vi "Setup Fast F Sweep.vi"(4 "TO, ms":u32=100, 5 "Retry on TO":bool, 7 "Generate F array":bool=TRUE, 8 "error in":errorcluster, 11 "RUS settings in":T1={"NI-DAQ lockin settings"={"Samples per sine wave"=0, "Sine waves per freq step"=0, "Output Representation"=enum."Real/Imaginary", "Low-pass filter"=enum."Butterworth", "Ranges and couplings "=[]}, "Fast swep settings"={"Update rate (Hz)"=250.0, "Start F, Hz"=200000.0, "Stop F"=1700000.0, "Number of points"=30000, "Amplitude"=2.1, "Init&amplitude"=TRUE, "IF"=1000.0, "Time constant"=0.1}, "Pre-sweep delay, s"=0.0, "Lockin mode"=enum."NI-DAQ", "SR Lockin"="GPIB0::10::INSTR", "DAQmx Device"="Dev3", "Clock Multiplier"=64, "Fast Sweep Data Out"={"DO clock task"="", "DO task"="", "Update clock task"="", "DAQ lockin task"="", "Pre-sweep counter task"=""}, "Lockin Range, V"=0.0, "F Array"=[], "Freq. update clock terminal"="", "DO Clock Rate (Hz)"=5000000.0, "ADC clock terminal"="/PFI4", "Pre-sweep counter terminal"="", "Samples per read"=10, "DO clock terminal"="", "Pre-sweep points"=0, "F points per write"=1000, "Total sweep time, s"=0.0, "Initial SYNTH phase"=0.0, "Record IF"=FALSE, "Save data settings"={"Save data"=TRUE, "Data Root Path"=path "", "File Prefix"="", "File Format"=enum."ASCII", "Save column names"=TRUE, "File Comments"="<Description of the current file>", "User/Prj"="<User Name/Project Description>"}, "Data file path"=path "", "New data user event"=refnum, "Stop user event"=refnum, "Number of channels"=1, "Auto-phase"=FALSE, "RP Transeiver"=refnum} {"Lockin Range, V" format="%#_6e"; "Fast swep settings"."IF" format="%#_6p"; "Fast swep settings"."Amplitude" min=0.0 max=2.5; "Fast swep settings"."Number of points" format="%.0p"; "Fast swep settings"."Stop F" format="%#_6p"; "Fast swep settings"."Start F, Hz" format="%#_6p"; "Fast swep settings"."Update rate (Hz)" format="%0.2f"; "NI-DAQ lockin settings"."Ranges and couplings"."Coupling" items=["default"=-1, "RSE"=10083, "NRSE"=10078, "Differential"=10106, "Pseudodifferential"=12529]}) -> (0 "error out":errorcluster, 1 "DO task setup time":u32, 3 "RUS settings out":T1={"NI-DAQ lockin settings"={"Samples per sine wave"=0, "Sine waves per freq step"=0, "Output Representation"=enum."Real/Imaginary", "Low-pass filter"=enum."Butterworth", "Ranges and couplings "=[]}, "Fast swep settings"={"Update rate (Hz)"=250.0, "Start F, Hz"=200000.0, "Stop F"=1700000.0, "Number of points"=30000, "Amplitude"=2.1, "Init&amplitude"=TRUE, "IF"=1000.0, "Time constant"=0.1}, "Pre-sweep delay, s"=0.0, "Lockin mode"=enum."NI-DAQ", "SR Lockin"="GPIB0::10::INSTR", "DAQmx Device"="Dev3", "Clock Multiplier"=64, "Fast Sweep Data Out"={"DO clock task"="", "DO task"="", "Update clock task"="", "DAQ lockin task"="", "Pre-sweep counter task"=""}, "Lockin Range, V"=0.0, "F Array"=[], "Freq. update clock terminal"="", "DO Clock Rate (Hz)"=5000000.0, "ADC clock terminal"="/PFI4", "Pre-sweep counter terminal"="", "Samples per read"=10, "DO clock terminal"="", "Pre-sweep points"=0, "F points per write"=1000, "Total sweep time, s"=0.0, "Initial SYNTH phase"=0.0, "Record IF"=FALSE, "Save data settings"={"Save data"=TRUE, "Data Root Path"=path "", "File Prefix"="", "File Format"=enum."ASCII", "Save column names"=TRUE, "File Comments"="<Description of the current file>", "User/Prj"="<User Name/Project Description>"}, "Data file path"=path "", "New data user event"=refnum, "Stop user event"=refnum, "Number of channels"=1, "Auto-phase"=FALSE, "RP Transeiver"=refnum} {"Lockin Range, V" format="%#_6e"; "Fast swep settings"."IF" format="%#_6p"; "Fast swep settings"."Amplitude" min=0.0 max=2.5; "Fast swep settings"."Number of points" format="%.0p"; "Fast swep settings"."Stop F" format="%#_6p"; "Fast swep settings"."Start F, Hz" format="%#_6p"; "Fast swep settings"."Update rate (Hz)" format="%0.2f"; "NI-DAQ lockin settings"."Ranges and couplings"."Coupling" items=["default"=-1, "RSE"=10083, "NRSE"=10078, "Differential"=10106, "Pseudodifferential"=12529]})   [LabVIEW 2016]
uses:
  Controls/Lockin mode.ctl
  NHMFL_Core/Libraries/Red Pitaya/RP Core/RP Transceiver/RP Transceiver.lvclass
  Controls/Sweep settings.ctl
  Controls/RUS NI-DAQ Lockin Settings.ctl
  Controls/RUS settings.ctl
  NHMFL_Core/Libraries/File/Controls/File formats.ctl
  NHMFL_Core/Libraries/File/Controls/Save data settings.ctl
panel:
  out "F1 out time":u32
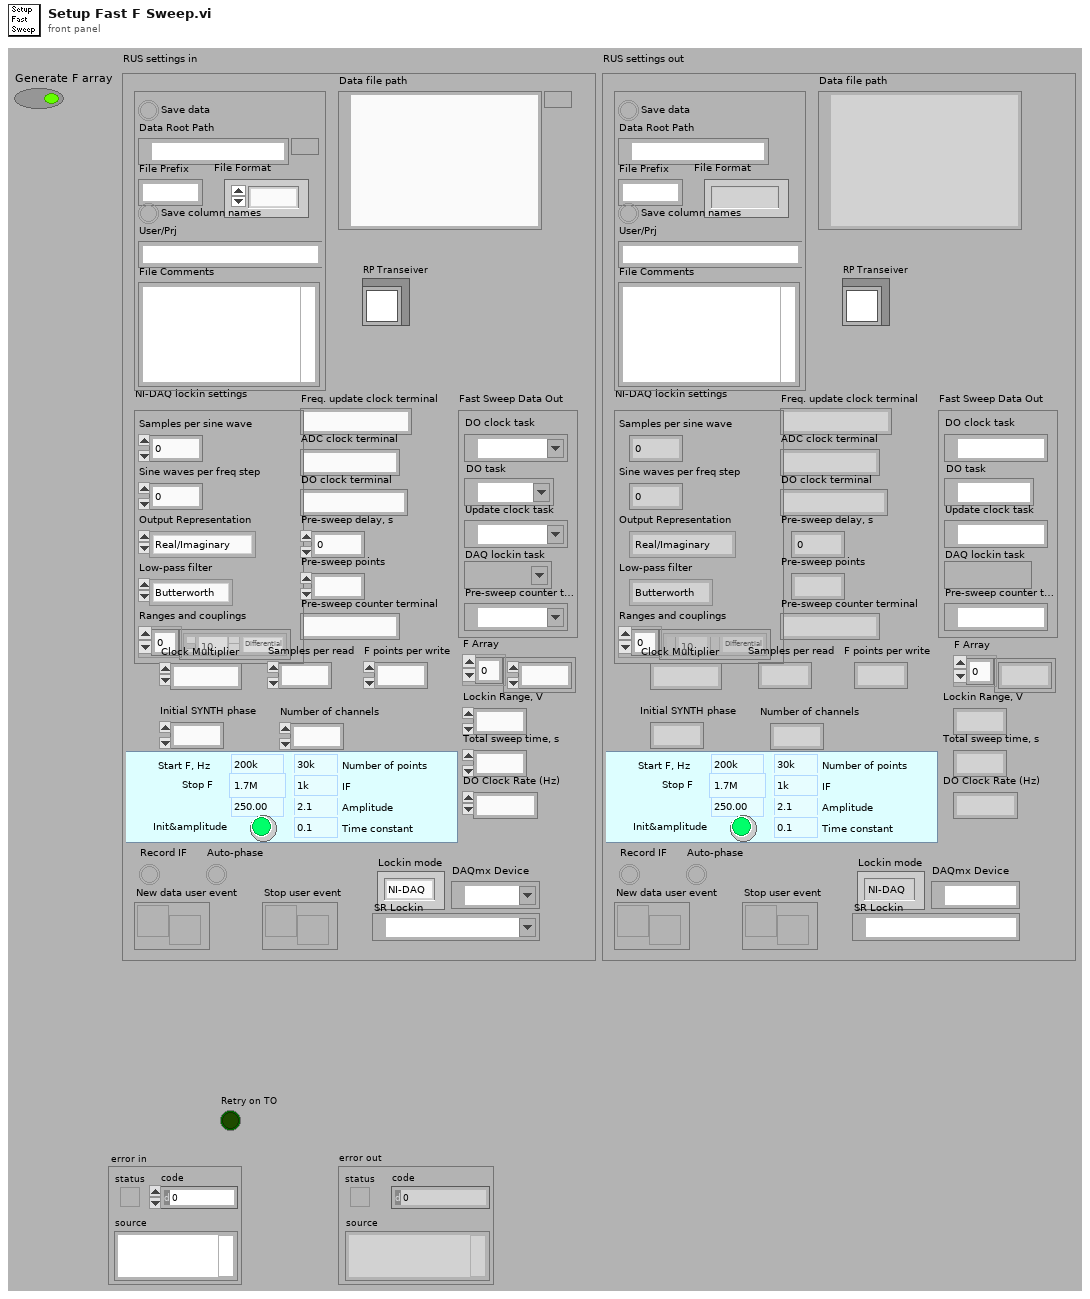
[diagram p1: front panel]
types:
  T1 = typedef "RUS settings.ctl" = cluster{"NI-DAQ lockin settings":T2, "Fast swep settings":T3, "Pre-sweep delay, s":dbl, "Lockin mode":T4, "SR Lockin":refnum<visa-resource-name>, "DAQmx Device":tag, "Clock Multiplier":i32, "Fast Sweep Data Out":cluster{"DO clock task":refnum<k21>, "DO task":refnum<k21>, "Update clock task":refnum<k21>, "DAQ lockin task":refnum<k21>, "Pre-sweep counter task":refnum<k21>}, "Lockin Range, V":sgl, "F Array":dbl[], "Freq. update clock terminal":string, "DO Clock Rate (Hz)":dbl, "ADC clock terminal":string, "Pre-sweep counter terminal":string, "Samples per read":i32, "DO clock terminal":string, "Pre-sweep points":i32, "F points per write":i32, "Total sweep time, s":dbl, "Initial SYNTH phase":dbl, "Record IF":bool, "Save data settings":T5, "Data file path":path, "New data user event":refnum<user-event>, "Stop user event":refnum<user-event>, "Number of channels":i32, "Auto-phase":bool, "RP Transeiver":refnum<class "RP Transceiver.lvclass">}
  T2 = typedef "RUS NI-DAQ Lockin Settings.ctl" = cluster{"Samples per sine wave":i32, "Sine waves per freq step":i32, "Output Representation":enum16{"Real/Imaginary", "Polar"}, "Low-pass filter":enum16{"No filtering", "Butterworth", "Bessel"}, "Ranges and couplings ":cluster{"Range":dbl, "Coupling":i32}[]}
  T3 = typedef "Sweep settings.ctl" = cluster{"Update rate (Hz)":dbl, "Start F, Hz":dbl, "Stop F":dbl, "Number of points":i32, "Amplitude":dbl, "Init&amplitude":bool, "IF":dbl, "Time constant":dbl}
  T4 = typedef "Lockin mode.ctl" = enum16{"SRS", "NI-DAQ", "Pitaya"}
  T5 = typedef "Save data settings.ctl" = cluster{"Save data":bool, "Data Root Path":path, "File Prefix":string, "File Format":T6, "Save column names":bool, "File Comments":string, "User/Prj":string}
  T6 = typedef "File formats.ctl" = enum16{"TDMS", "ASCII", "BINARY"}
  T7 = enum16{"Direct, clock*f1", "Direct, clock*f2", "Heterodyne"}
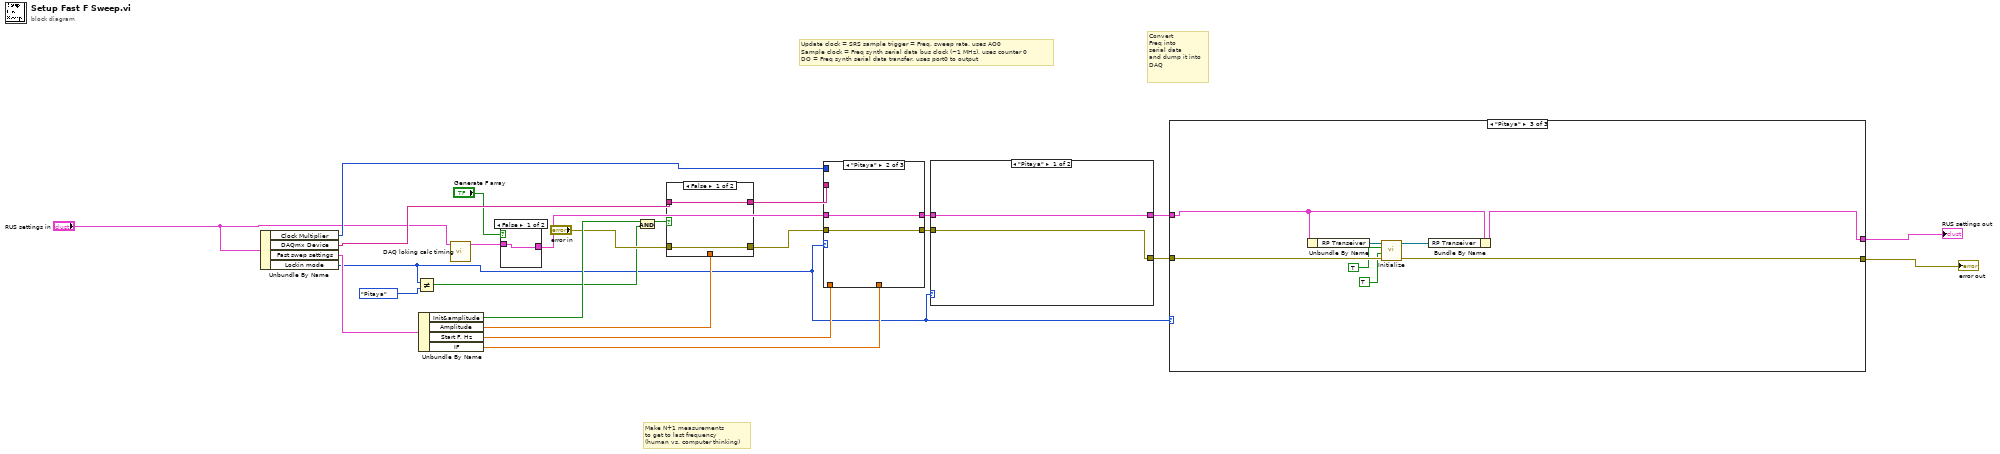
[diagram p0: block diagram]
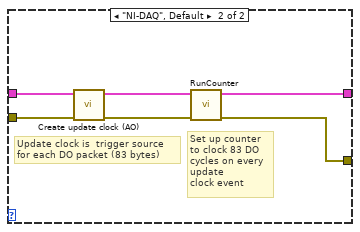
[diagram p2: hidden frame]
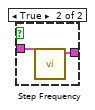
[diagram p3: hidden frame]
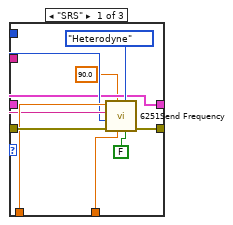
[diagram p4: hidden frame]
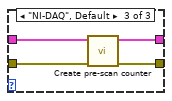
[diagram p5: hidden frame]
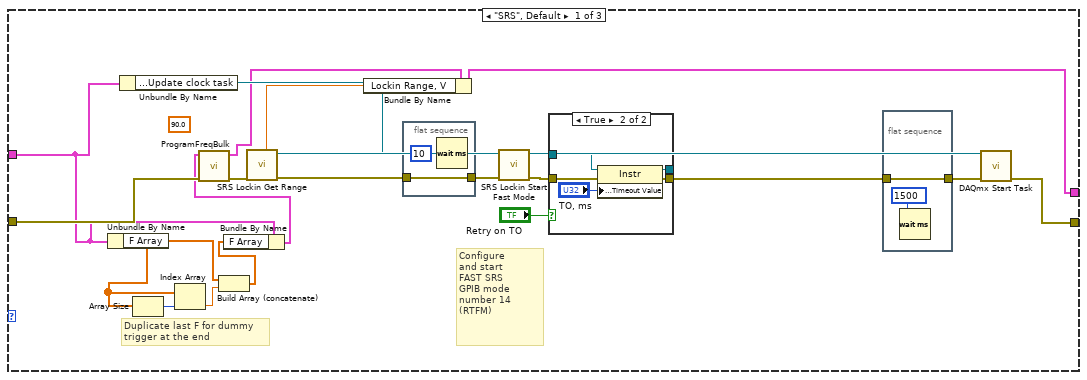
[diagram p6: hidden frame]
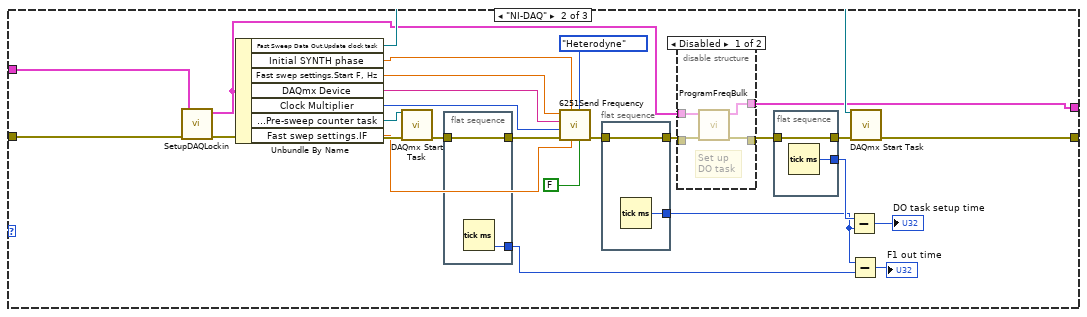
[diagram p8: hidden frame]
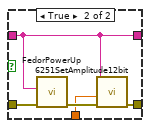
[diagram p10: hidden frame]
diagram:
  # "Make N+1 measurements\nto get to last frequency\n(human vs. computer thinking)"
  # "Convert \nFreq into \nserial data \nand dump it into \nDAQ"
  # "Update clock = SRS sample trigger = Freq. sweep rate, uses AO0\nSample clock = Freq synth serial data bus clock (~1 MHz), uses counter 0\nDO = Freq synth serial data transfer, uses port0 to output"
  n1 = Unbundle By Name("RUS settings in") -> ("Clock Multiplier"=w13:i32, "DAQmx Device"=w15:tag, "Fast swep settings"=w16:T3, "Lockin mode"=w1:T4)
  n2 = Not Equal?(x=w1, y=Lockin_mode."Pitaya" ("Lockin mode")) -> (x != y?=w2:bool)
  n3 = Unbundle By Name(w16) -> ("Init&amplitude"=w23:bool, "Amplitude"=w24:dbl, "Start F, Hz"=w11:dbl, "IF"=w19:dbl)
  n4 = call "DAQ loking calc timing.vi"("RUS settings"="RUS settings in") -> ("RUS settings out"=w9:T1)  [unwired: 10 in]
  n5 = case shown="False" "Generate F array" {
    tunnel: w9 -> [w25 w27]
    tunnel: [w25 w26] -> w7
    frame False {
    }
    frame True {
      n6 = call "Step Frequency.vi"("RUS settings"=w27) -> ("RUS settings out"=w26:T1)  [unwired: 3 in, 7 out]
    }
  }
  n7 = And(x=w23, y=w2) -> (x .and. y?=w3:bool)
  n8 = case shown="False" w3 {
    tunnel: "error in" -> [w29 w34]
    tunnel: [w29 w32] -> w21
    tunnel: w15 -> [w28 w31]
    tunnel: [w28 w31] -> w20
    tunnel: w24 -> [_ w30]
    frame False {
    }
    frame True {
      n9 = call "FedorPowerUp.vi"("error in (no error)"=w34, "DAQmx Device Name"=w31) -> ("error out"=w33:errorcluster)  [unwired: 9 out]
      n10 = call "6251SetAmplitude12bit.vi"("error in (no error)"=w33, "0 to 2.1 VRMS"=w30, "DAQmx Device Name"=w31) -> ("error out"=w32:errorcluster)  [unwired: 8 out]
    }
  }
  n11 = case shown="\"Pitaya\"" w1 {
    tunnel: w21 -> [w44 w46 w50]
    tunnel: [w43 w46 w49] -> w8
    tunnel: w19 -> [w42 _ _]
    tunnel: w11 -> [w40 _ _]
    tunnel: w20 -> [w39 _ _]
    tunnel: w13 -> [w38 _ _]
    tunnel: w7 -> [w36 w45 w48]
    tunnel: [w36 w45 w47] -> w6
    frame "SRS" {
      n12 = call "6251Send Frequency.vi"("Use hardware clock for DO"=FALSE ("6251"), "Mode"=T7."Heterodyne", "IF (Hz)"=w42, "Phase (degrees)"=90.0, "error in (no error)"=w44, "Clock Multiplier"=w38, "DAQmx Device Name"=w39, "f (Hz)"=w40) -> ("error out"=w43:errorcluster)  [unwired: 2 in, 1 out]
    }
    frame "Pitaya" {
    }
    frame "NI-DAQ", Default {
      n13 = call "Create pre-scan counter.vi"("error in"=w50, "RUS settings"=w48) -> ("error out"=w49:errorcluster, "RUS settings out"=w47:T1)  [unwired: 8 in]
    }
  }
  n14 = case shown="\"Pitaya\"" w1 {
    tunnel: [w51 w57] -> w18
    tunnel: [w52 w55] -> w14
    tunnel: w8 -> [w51 w54]
    tunnel: w6 -> [w52 w53]
    frame "Pitaya" {
    }
    frame "NI-DAQ", Default {
      # "Set up counter\nto clock 83 DO\ncycles on every\nupdate \nclock event"
      # "Update clock is  trigger source\nfor each DO packet (83 bytes)"
      n15 = call "Create update clock (AO).vi"("error in"=w54, "RUS settings"=w53) -> ("error out"=w58:errorcluster, "RUS settings out"=w56:T1)  [unwired: 3 in, 5 out]
      n16 = call "RunCounter.vi"("error in (no error)"=w58, "RUS settings"=w56) -> ("error out"=w57:errorcluster, "RUS settings out"=w55:T1)  [unwired: 2 in, 6 out]
    }
  }
  n17 = case shown="\"Pitaya\"" w1 {
    tunnel: w18 -> [w66 w116 w132]
    tunnel: [w70 w102 w131] -> w17
    tunnel: w14 -> [w61 w91 w136]
    tunnel: [w68 w97 w134] -> w10
    frame "SRS", Default {
      (unwired) 90.0 ("Phase (degrees)")
      # "Duplicate last F for dummy \ntrigger at the end"
      # "Configure \nand start \nFAST SRS\nGPIB mode\nnumber 14\n(RTFM)"
      n18 = Unbundle By Name(w61) -> ("F Array"=w62:dbl[])
      n19 = Unbundle By Name(w61) -> ("Fast Sweep Data Out.Update clock task"=w69:refnum<k21>)
      n20 = Array Size(array=w62) -> (size(s)=w63:i32)
      n21 = Index Array(array=w62, index=w63) -> (element=w64:dbl)
      n22 = Build Array (concatenate)(w62, w64) -> (w60:dbl[])
      n23 = Bundle By Name(cluster=w61, "F Array"=w60) -> (w59:T1)
      n24 = call "ProgramFreqBulk.vi"("error in (no error)"=w66, "RUS settings"=w59) -> ("error out"=w73:errorcluster, "RUS settings out"=w65:T1)  [unwired: 3 in, 5 out]
      n25 = call "SRS Lockin Get Range.vi"("error in (no error)"=w73) -> ("error out"=w75:errorcluster, "VISA resource name out"=w79:refnum<visa-resource-name>, "Range, V"=w67:sgl)  [unwired: 1 in, 7 out]
      n26 = Bundle By Name(cluster=w65, "Lockin Range, V"=w67) -> (w68:T1)
      n27 = flat-sequence {
        tunnel: w75 -> [w83]
        tunnel: [w83] -> w74
        frame #0 {
          n28 = Wait (ms)(milliseconds to wait=u32 10) -> ()  [unwired: 1 out]
        }
      }
      n29 = call "SRS Lockin Start Fast Mode.vi"("error in (no error)"=w74, "VISA Resource Name"=w79) -> ("error out"=w78:errorcluster, "VISA resource name out"=w76:refnum<visa-resource-name>)  [unwired: 1 in, 7 out]
      n30 = case shown="True" "Retry on TO" {
        tunnel: w78 -> [w85 w90]
        tunnel: [w85 w89] -> w72
        tunnel: w76 -> [w84 w87]
        tunnel: [w84 w86] -> _
        frame False {
        }
        frame True {
          n31 = property class="Instr"(reference=w87, error in=w90, "General Settings:Timeout Value"="TO, ms") -> (reference out=w86:refnum<visa-resource-name>, error out=w89:errorcluster)
        }
      }
      n32 = flat-sequence {
        tunnel: w72 -> [w81]
        tunnel: [w81] -> w71
        frame #0 {
          n33 = Wait (ms)(milliseconds to wait=u32 1500) -> ()  [unwired: 1 out]
        }
      }
      n34 = call <vilib>:"DAQmx Start Task.vi"("task/channels in"=w69, "error in"=w71) -> ("error out"=w70:errorcluster)  [unwired: 13 out]
    }
    frame "NI-DAQ" {
      n35 = call "SetupDAQLockin.vi"("error in (no error)"=w116, "RUS settings"=w91) -> ("error out"=w103:errorcluster, "RUS settings out"=w98:T1)  [unwired: 8 in]
      n36 = Unbundle By Name(w98) -> ("Fast Sweep Data Out.Update clock task"=w101:refnum<k21>, "Initial SYNTH phase"=w92:dbl, "Fast swep settings.Start F, Hz"=w95:dbl, "DAQmx Device"=w100:tag, "Clock Multiplier"=w94:i32, "Fast Sweep Data Out.Pre-sweep counter task"=w104:refnum<k21>, "Fast swep settings.IF"=w96:dbl)
      n37 = call <vilib>:"DAQmx Start Task.vi"("task/channels in"=w104, "error in"=w103) -> ("error out"=w109:errorcluster)  [unwired: 13 out]
      n38 = flat-sequence {
        tunnel: w109 -> [w124]
        tunnel: [w124] -> w108
        tunnel: [w123] -> w106
        frame #0 {
          n39 = Tick Count (ms)() -> (millisecond timer value=w123:u32)
        }
      }
      n40 = call "6251Send Frequency.vi"("Use hardware clock for DO"=FALSE ("6251"), "Mode"=T7."Heterodyne", "IF (Hz)"=w96, "Phase (degrees)"=w92, "error in (no error)"=w108, "Clock Multiplier"=w94, "DAQmx Device Name"=w100, "f (Hz)"=w95) -> ("error out"=w113:errorcluster)  [unwired: 2 in, 1 out]
      n41 = flat-sequence {
        tunnel: w113 -> [w128]
        tunnel: [w128] -> w99
        tunnel: [w127] -> w93
        frame #0 {
          n42 = Tick Count (ms)() -> (millisecond timer value=w127:u32)
        }
      }
      n43 = disable-structure shown="Disabled" {
        disable-tunnel: [w120 w121] -> w112
        disable-tunnel: w99 -> [w119 w121]
        disable-tunnel: w98 -> [w118 w122]
        disable-tunnel: [w117 w122] -> w97
        frame Disabled {
          # "Set up\nDO task"
          n44 = call "ProgramFreqBulk.vi"("error in (no error)"=w119, "RUS settings"=w118) -> ("error out"=w120:errorcluster, "RUS settings out"=w117:T1)  [unwired: 3 in, 5 out]
        }
        frame Enabled {
        }
      }
      n45 = flat-sequence {
        tunnel: w112 -> [w126]
        tunnel: [w126] -> w111
        tunnel: [w125] -> w107
        frame #0 {
          n46 = Tick Count (ms)() -> (millisecond timer value=w125:u32)
        }
      }
      n47 = Subtract(x=w107, y=w93) -> (x-y=→"DO task setup time":u32)
      n48 = Subtract(x=w93, y=w106) -> (x-y=→"F1 out time":u32)
      n49 = call <vilib>:"DAQmx Start Task.vi"("task/channels in"=w101, "error in"=w111) -> ("error out"=w102:errorcluster)  [unwired: 12 in, 1 out]
    }
    frame "Pitaya" {
      n50 = Unbundle By Name(w136) -> ("RP Transeiver"=w135:refnum<class "RP Transceiver.lvclass">)
      n51 = call-dynamic "Initialize.vi"("error in (no error)"=w132, "Send \"Connect client\""=TRUE ("Send \"Connect client\""), "Reset"=TRUE, "RP Transceiver in"=w135) -> ("error out"=w131:errorcluster, "RP Transceiver out"=w133:refnum<class "RP Transceiver.lvclass">)  [unwired: 6 in]
      n52 = Bundle By Name(cluster=w136, "RP Transeiver"=w133) -> (w134:T1)
    }
  }
  "error out" <- w17
  "RUS settings out" <- w10
